vi "Desktop Main.vi"() -> ()   [LabVIEW 2021]
doc: "Demonstrates the use of Transmission Control Protocol (TCP) to continuously send LED status to the myRIO target."
panel:
  out "Tank":dbl(slide) scale=0.0..10.0
  out "error out":errorcluster
  in  "Stop":bool
  # "Overview: Demonstrates the use of Transmission Control Protocol (TCP) to continuously send LED status to the myRIO target.\nInstructions:\n1. Run this VI\n2. Open RT Main.vi and follow its front panel instructions. \n3. Click Stop to stop this VI. Stopping this VI also terminates the running of RT Main.vi."
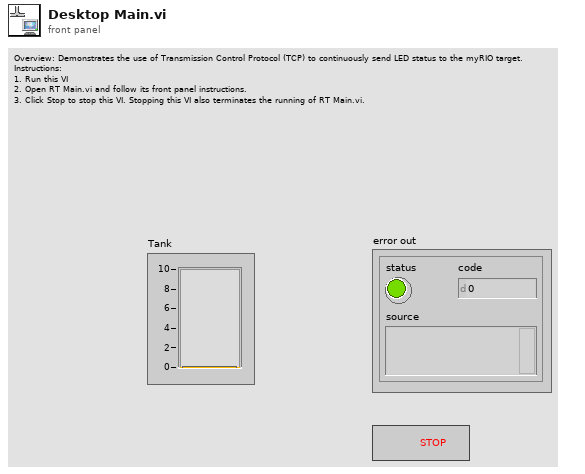
[diagram p1: front panel]
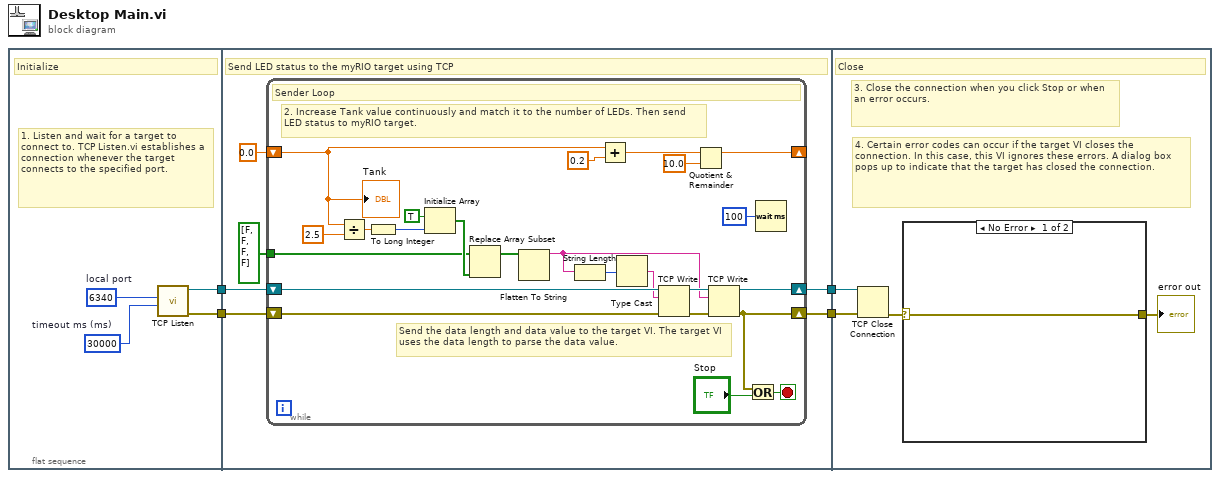
[diagram p0: block diagram]
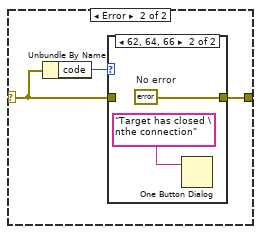
[diagram p2: hidden frame]
diagram:
  n1 = flat-sequence {
    tunnel: [w7] -> w2
    tunnel: [w6] -> w1
    tunnel: [w14] -> w4
    tunnel: [w13] -> w3
    tunnel: w2 -> [w12]
    tunnel: w1 -> [w11]
    tunnel: w4 -> [w42]
    tunnel: w3 -> [w41]
    frame #0 {
      w5 = 30000  # timeout ms (ms)
      w8 = u16 6340  # local port
      # "1. Listen and wait for a target to connect to. TCP Listen.vi establishes a connection whenever the target connects to the specified port."
      # "Initialize"
      n2 = call <vilib>:"TCP Listen.vi"("timeout ms (wait forever: -1)"=w5, "port"=w8) -> ("error out"=w6:errorcluster, "connection ID"=w7:refnum<k5>)  [unwired: 5 in, 3 out]
    }
    frame #1 {
      # "Send LED status to the myRIO target using TCP"
      n3 = while {
        shift-right: [w33] -> w14
        shift-left: w12 -> [w34]
        shift-right: [w32] -> w13
        shift-left: w11 -> [w20]
        shift-right: [w22] -> _
        shift-left: 0.0 ("y") -> [w26]
        tunnel: bool[] [FALSE, FALSE, FALSE, FALSE] -> [w16]
        stop <- w37 stop-if-true
        # "2. Increase Tank value continuously and match it to the number of LEDs. Then send LED status to myRIO target."
        # "Send the data length and data value to the target VI. The target VI uses the data length to parse the data value."
        # "Sender Loop"
        n4 = Divide(x=w26, y=2.5) -> (x/y=w30:dbl)
        n5 = To Long Integer(number=w30) -> (32bit integer=w19:i32)
        n6 = Initialize Array(TRUE ("element"), w19) -> (w17:bool[])
        n7 = Replace Array Subset(array=w16, new element=w17) -> (w15:bool[])  [unwired: 1 in]
        n8 = Flatten To String(anything=w15) -> (data string=w24:string)  [unwired: 3 in, 2 out]
        n9 = String Length(string=w24) -> (length=w25:i32)
        n10 = Add(x=w26, y=0.2) -> (x+y=w27:dbl)
        n11 = Type Cast(x=w25) -> (*(type *) &x=w23:string)  [unwired: 1 out]
        n12 = TCP Write(connection ID=w34, data in=w23, error in (no error)=w20) -> (connection ID out=w35:refnum<k5>, error out=w36:errorcluster)  [unwired: 1 in, 1 out]
        n13 = Quotient & Remainder(x=w27, y=10.0) -> (x-y*floor(x/y)=w22:dbl)  [unwired: 1 out]
        n14 = TCP Write(connection ID=w35, data in=w24, error in (no error)=w36) -> (connection ID out=w33:refnum<k5>, error out=w32:errorcluster)  [unwired: 1 in, 1 out]
        n15 = Or(x=w32, y="Stop") -> (x .or. y?=w37:bool)
        n16 = Wait (ms)(milliseconds to wait=u32 100) -> ()  [unwired: 1 out]
        "Tank" <- w26
      }
    }
    frame #2 {
      # "4. Certain error codes can occur if the target VI closes the connection. In this case, this VI ignores these errors. A dialog box pops up to indicate that the target has closed the connection."
      # "3. Close the connection when you click Stop or when an error occurs."
      # "Close"
      n17 = TCP Close Connection(connection ID=w42, error in (no error)=w41) -> (error out=w40:errorcluster)  [unwired: 2 out]
      n18 = case shown="No Error" w40 {
        selector: w40 -> [w43 w44]
        tunnel: [w43 w45] -> w39
        frame No Error {
        }
        frame Error {
          n19 = Unbundle By Name(w44) -> ("code"=w46:i32)
          n20 = case shown="62, 64, 66" w46 {
            tunnel: w44 -> [w47 _]
            tunnel: [w47 w48] -> w45
            frame Default {
            }
            frame 62, 64, 66 {
              w48 = errorcluster {"status"=FALSE, "code"=0, "source"=""}  # No error
              n21 = One Button Dialog(message="Target has closed \nthe connection") -> ()  [unwired: 1 in, 1 out]
            }
          }
        }
      }
      "error out" <- w39
    }
  }
